vi "Add Initialization Block Diagram Content.vi"(8 "error in (no error)":errorcluster, 10 "Init":T1, 11 "EST Output in":refnum<class "EST Output.lvclass">) -> (0 "error out":errorcluster, 3 "EST Output out":refnum<class "EST Output.lvclass">)   [LabVIEW 2015, in "EST Output.lvclass"]
uses:
  EST Output.lvclass
  VI/VI/Init.Refs.ctl
  <vilib>/Utility/miscctls.llb/LVPointTypeDef.ctl
  <vilib>/_script/New VI Object TypeDefs/NewVIObject_LVRelativePositionTypeDef.ctl
  <vilib>/_script/New VI Object TypeDefs/NewVIObject_LVRelativeDirectionTypeDef.ctl
  <vilib>/Utility/miscctls.llb/LVPoint32TypeDef.ctl
  EST Output.lvclass/EST Output.ctl
  Signal/Read Signal Name.vi
  Read Memory Template Path.vi
  Read Load Path.vi
  VI/Structures/Structures.lvclass
  VI/VI/VI.lvclass
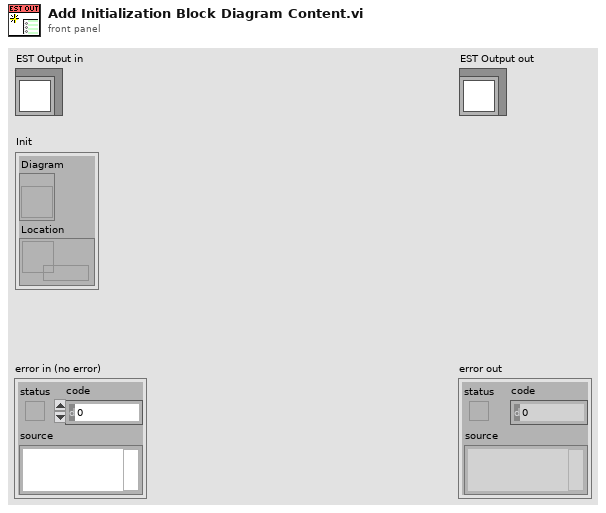
[diagram p1: front panel]
types:
  T1 = typedef "VI.lvclass/Init.Refs.ctl" = cluster{"Diagram":refnum<vi>, "Location":refnum<data-value>}
  T2 = typedef "NewVIObject_LVRelativePositionTypeDef.ctl" = cluster{"Refnum":refnum<vi>, "Relative Direction":T3, "Point32":T4}
  T3 = typedef "NewVIObject_LVRelativeDirectionTypeDef.ctl" = enum32{"Right", "Left", "Top", "Bottom", "Top Right", "Top Left", "Bottom Right", "Bottom Left"}
  T4 = typedef "LVPoint32TypeDef.ctl" = cluster{"Horizontal":i32, "Vertical":i32}
  T5 = typedef "LVPointTypeDef.ctl" = cluster{"Horizontal":i16, "Vertical":i16}
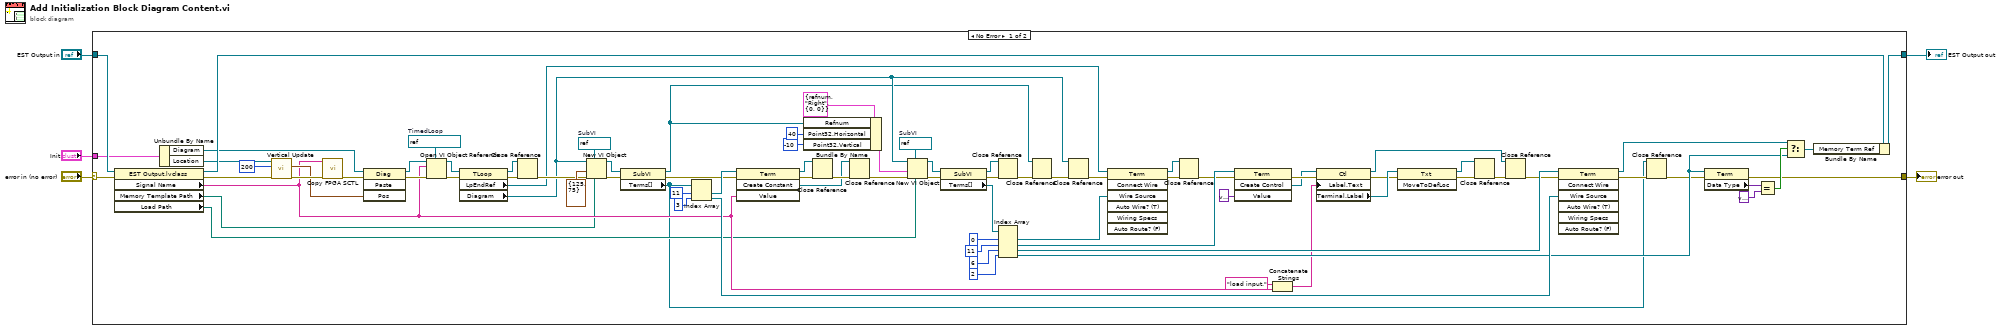
[diagram p0: block diagram]
diagram:
  n1 = case shown="No Error" "error in (no error)" {
    selector: "error in (no error)" -> [w44 w91]
    tunnel: "EST Output in" -> [w51 w92]
    tunnel: [w50 w91] -> w3
    tunnel: [w47 w92] -> w2
    tunnel: "Init" -> [w46 _]
    frame No Error {
      w36 = refnum<vi> refnum  # TimedLoop
      w81 = refnum<vi> refnum  # SubVI
      w76 = refnum<vi> refnum  # SubVI
      n2 = property class="EST Output.lvclass"(reference=w51, error in=w44) -> (reference out=w49:refnum<class "EST Output.lvclass">, error out=w26:errorcluster, "Signal Name"=w31:string, "Memory Template Path"=w23:path, "Load Path"=w24:path)
      n3 = Unbundle By Name(w46) -> ("Diagram"=w40:refnum<vi>, "Location"=w25:refnum<data-value>)
      n4 = call "Vertical Update.vi"("error in (no error)"=w26, "Vertical Change"=i16 200, "Location"=w25) -> ("error out"=w39:errorcluster, "location out"=w37:T5)  [unwired: 6 in, 1 out]
      n5 = call "Copy FPGA SCTL.vi"("error in (no error)"=w39, "SCTL Name"=w31) -> ("error out"=w38:errorcluster)  [unwired: 9 in]
      n6 = invoke class="Diag" method="Paste"(reference=w40, error in=w38, "Pos"=w37) -> (reference out=w35:refnum<vi>, error out=w34:errorcluster)  [unwired: 1 in, 2 out]
      n7 = Open VI Object Reference(7:w36, 8:w34, 10:w31, 11:w35) -> (0:w33:errorcluster, 3:w32:refnum<vi>)
      n8 = property class="TLoop"(reference=w32, error in=w33) -> (reference out=w73:refnum<vi>, error out=w75:errorcluster, "LpEndRef"=w72:refnum<vi>, "Diagram"=w9:refnum<vi>)
      n9 = Close Reference(reference=w73, error in (no error)=w75) -> (error out=w74:errorcluster)
      n10 = New VI Object(vi object class=w76, owner refnum=w9, position/next to=T5 {"Horizontal"=125, "Vertical"=75} ("location"), 6:w23, 8:w74) -> (object refnum=w79:refnum<vi>, 0:w80:errorcluster)  [unwired: 3 in]
      n11 = property class="SubVI"(reference=w79, error in=w80) -> (reference out=w8:refnum<vi>, error out=w12:errorcluster, "Terms[]"=w14:refnum<vi>[])
      n12 = Index Array(array=w14, index #1=11 ("index"), index #2=3 ("index")) -> (element #1=w70:refnum<vi>, element #2=w71:refnum<vi>)
      n13 = invoke class="Term" method="Create Constant"(reference=w70, error in=w12, "Value"=w31) -> (reference out=w69:refnum<vi>, error out=w68:errorcluster, "Create Constant"=w65:refnum<vi>)  [unwired: 1 in, 1 out]
      n14 = Bundle By Name(cluster=T2 {"Refnum"=refnum, "Relative Direction"=enum."Right", "Point32"={"Horizontal"=0, "Vertical"=0}} ("Relative Position"), "Refnum"=w8, "Point32.Horizontal"=40, "Point32.Vertical"=-10) -> (w29:T2)
      n15 = Close Reference(reference=w69, error in (no error)=w68) -> (error out=w67:errorcluster)
      n16 = Close Reference(reference=w65, error in (no error)=w67) -> (error out=w66:errorcluster)
      n17 = New VI Object(vi object class=w81, owner refnum=w9, position/next to=w29, 6:w24, 8:w66) -> (object refnum=w83:refnum<vi>, 0:w82:errorcluster)  [unwired: 3 in]
      n18 = property class="SubVI"(reference=w83, error in=w82) -> (reference out=w64:refnum<vi>, error out=w63:errorcluster, "Terms[]"=w86:refnum<vi>[])
      n19 = Close Reference(reference=w64, error in (no error)=w63) -> (error out=w13:errorcluster)
      n20 = Index Array(array=w86, index #1=0 ("index"), index #2=11 ("index"), index #3=6 ("index"), index #4=2 ("index")) -> (element #1=w62:refnum<vi>, element #2=w61:refnum<vi>, element #3=w60:refnum<vi>, element #4=w54:refnum<vi>)
      n21 = Close Reference(reference=w8, error in (no error)=w13) -> (error out=w11:errorcluster)
      n22 = Close Reference(reference=w9, error in (no error)=w11) -> (error out=w10:errorcluster)
      n23 = invoke class="Term" method="Connect Wire"(reference=w72, error in=w10, "Wire Source"=w62) -> (reference out=w19:refnum<vi>, error out=w18:errorcluster)  [unwired: 4 in, 5 out]
      n24 = Close Reference(reference=w19, error in (no error)=w18) -> (error out=w17:errorcluster)
      n25 = invoke class="Term" method="Create Control"(reference=w61, error in=w17, "Value"=variant) -> (error out=w88:errorcluster, "Create Control"=w87:refnum<vi>)  [unwired: 1 in, 2 out]
      n26 = Concatenate Strings("load input." ("string"), w31) -> (w7:string)
      n27 = property class="Ctl"(reference=w87, error in=w88, "Label.Text"=w7) -> (reference out=w43:refnum<vi>, error out=w41:errorcluster, "Terminal.Label"=w42:refnum<vi>)
      n28 = invoke class="Txt" method="MoveToDefLoc"(reference=w42, error in=w41) -> (reference out=w22:refnum<vi>, error out=w20:errorcluster)  [unwired: 1 in, 1 out]
      n29 = Close Reference(reference=w22, error in (no error)=w20) -> (error out=w21:errorcluster)
      n30 = Close Reference(reference=w43, error in (no error)=w21) -> (error out=w59:errorcluster)
      n31 = invoke class="Term" method="Connect Wire"(reference=w60, error in=w59, "Wire Source"=w71) -> (reference out=w53:refnum<vi>, error out=w16:errorcluster)  [unwired: 4 in, 5 out]
      n32 = Close Reference(reference=w14, error in (no error)=w16) -> (error out=w15:errorcluster)
      n33 = property class="Term"(reference=w54, error in=w15) -> (error out=w50:errorcluster, "Data Type"=w57:variant)  [unwired: 1 out]
      n34 = Equal?(x=w57, y=variant ("x")) -> (x = y?=w55:bool)
      n35 = Select(t=w53, s=w55, f=w54) -> (s? t:f=w48:refnum<vi>)
      n36 = Bundle By Name(cluster=w49, "Memory Term Ref"=w48) -> (w47:refnum<class "EST Output.lvclass">)
    }
    frame Error {
    }
  }
  "error out" <- w3
  "EST Output out" <- w2
